vi "TEST - Filter 1D Array.vi"(8 "error in (no error)":errorcluster) -> (0 "error out":errorcluster, 2 "Pass?":bool)   [LabVIEW 2009]
doc: "This VI template can be used for the functional testing of VIs; this implementation includes handling for the testing of polymorphic VIs, and the polymorphic elements should be removed if not needed.\n\nCoded by Douglas A. Femec, January 24, 2006.\n\nCopyright (c) 2005-2006 MKS Instruments, Inc.\nAll rights reserved."
uses:
  TEST - Filter 1D Array - Inputs.ctl
  Polymorphizer+ Data Type.ctl
  TEST - Filter 1D Array - Outputs.ctl
  source/library/Filter 1D Array/Filter 1D Array (EXT).vi
  source/library/Filter 1D Array/Filter 1D Array with Scalar (EXT).vi
  source/library/Filter 1D Array/Filter 1D Array (DBL).vi
  source/library/Filter 1D Array/Filter 1D Array with Scalar (DBL).vi
  source/library/Filter 1D Array/Filter 1D Array with Scalar (LVObject).vi
  source/library/Filter 1D Array/Filter 1D Array (LVObject).vi
  source/library/Filter 1D Array/Filter 1D Array (I64).vi
  source/library/Filter 1D Array/Filter 1D Array with Scalar (I64).vi
  source/library/Filter 1D Array/Filter 1D Array (U64).vi
  source/library/Filter 1D Array/Filter 1D Array with Scalar (U64).vi
  source/library/Filter 1D Array/Filter 1D Array (SGL).vi
  source/library/Filter 1D Array/Filter 1D Array with Scalar (SGL).vi
  source/library/Filter 1D Array/Filter 1D Array (I32).vi
  source/library/Filter 1D Array/Filter 1D Array with Scalar (I32).vi
  source/library/Filter 1D Array/Filter 1D Array (I16).vi
  source/library/Filter 1D Array/Filter 1D Array with Scalar (I16).vi
  source/library/Filter 1D Array/Filter 1D Array (I8).vi
  source/library/Filter 1D Array/Filter 1D Array with Scalar (I8).vi
  source/library/Filter 1D Array/Filter 1D Array (U32).vi
  source/library/Filter 1D Array/Filter 1D Array with Scalar (U32).vi
  source/library/Filter 1D Array/Filter 1D Array (U16).vi
  source/library/Filter 1D Array/Filter 1D Array with Scalar (U16).vi
  source/library/Filter 1D Array/Filter 1D Array (U8).vi
  source/library/Filter 1D Array/Filter 1D Array with Scalar (U8).vi
  source/library/Filter 1D Array/Filter 1D Array (CXT).vi
  source/library/Filter 1D Array/Filter 1D Array with Scalar (CXT).vi
  source/library/Filter 1D Array/Filter 1D Array (CDB).vi
  source/library/Filter 1D Array/Filter 1D Array with Scalar (CDB).vi
  source/library/Filter 1D Array/Filter 1D Array (CSG).vi
  source/library/Filter 1D Array/Filter 1D Array with Scalar (CSG).vi
  source/library/Filter 1D Array/Filter 1D Array (Boolean).vi
  source/library/Filter 1D Array/Filter 1D Array with Scalar (Boolean).vi
  source/library/Filter 1D Array/Filter 1D Array (String).vi
  source/library/Filter 1D Array/Filter 1D Array with Scalar (String).vi
  source/library/Filter 1D Array/Filter 1D Array (Path).vi
  source/library/Filter 1D Array/Filter 1D Array with Scalar (Path).vi
  source/library/Filter 1D Array/Filter 1D Array (Variant).vi
  source/library/Filter 1D Array/Filter 1D Array with Scalar (Variant).vi
  TestClass/TestClass.lvclass
panel:
  out "Generated Outputs":T1[][](array[typedef]) {"Filtered Array (Scalar)" format="%.2f"; "Filtered Array" format="%.2f"}
  in  "Expected Outputs":T1[](array[typedef])=[{"Description"="Expect empty array", "Filtered Array"=[], "Filtered Array (Scalar)"=[]}, {"Description"="Expect no elements filtered", "Filtered Array"=[0.0, 0.0, 0.0, 0.0], "Filtered Array (Scalar)"=[0.0, 0.0, 0.0, 0.0]}, {"Description"="Expect some elements filtered", "Filtered Array"=[0.0, 0.0], "Filtered Array (Scalar)"=[0.0, 0.0]}, {"Description"="Expect all elements filtered", "Filtered Array"=[], "Filtered Array (Scalar)"=[1.0, 1.0]}, {"Description"="Expect all elements filtered", "Filtered Array"=[], "Filtered Array (Scalar)"=[1.0, 1.0]}, {"Description"="Expect all elements filtered", "Filtered Array"=[], "Filtered Array (Scalar)"=[1.0, 1.0]}, {"Description"="Expect all elements filtered", "Filtered Array"=[], "Filtered Array (Scalar)"=[1.0, 1.0]}, {"Description"="Expect all elements filtered", "Filtered Array"=[], "Filtered Array (Scalar)"=[1.0, 1.0]}, {"Description"="Expect all elements filtered", "Filtered Array"=[], "Filtered Array (Scalar)"=[1.0, 1.0]}, {"Description"="Expect all elements filtered", "Filtered Array"=[], "Filtered Array (Scalar)"=[]}, {"Description"="Expect some elements filtered", "Filtered Array"=[0.0, 0.0], "Filtered Array (Scalar)"=[1.0, 1.0]}, {"Description"="Expect some elements filtered", "Filtered Array"=[1.0, 1.0], "Filtered Array (Scalar)"=[1.0, 1.0]}] {"Filtered Array (Scalar)" format="%.2f"; "Filtered Array" format="%.2f"}
  in  "Inputs":T2[](array[typedef])=[{"Description"="Empty arrays", "Data Types to Test"=[enum."EXT", enum."DBL", enum."SGL", enum."I32", enum."I16", enum."I8", enum."U32", enum."U16", enum."U8", enum."CXT", enum."CDB", enum."CSG", enum."Boolean", enum."String", enum."Path", enum."Variant", enum."I64", enum."U64", enum."LabVIEW Object"], "Array"=[], "Items to Filter"=[], "Scalar Item to Filter"=0.0}, {"Description"="No element to filter", "Data Types to Test"=[enum."EXT", enum."DBL", enum."SGL", enum."I32", enum."I16", enum."I8", enum."U32", enum."U16", enum."U8", enum."CXT", enum."CDB", enum."CSG", enum."Boolean", enum."String", enum."Path", enum."Variant", enum."I64", enum."U64", enum."LabVIEW Object"], "Array"=[0.0, 0.0, 0.0, 0.0], "Items to Filter"=[1.0], "Scalar Item to Filter"=1.0}, {"Description"="Filter some elements", "Data Types to Test"=[enum."EXT", enum."DBL", enum."SGL", enum."I32", enum."I16", enum."I8", enum."U32", enum."U16", enum."U8", enum."CXT", enum."CDB", enum."CSG", enum."Boolean", enum."String", enum."Path", enum."Variant", enum."I64", enum."U64", enum."LabVIEW Object"], "Array"=[0.0, 1.0, 0.0, 1.0], "Items to Filter"=[1.0], "Scalar Item to Filter"=1.0}, {"Description"="Filter all elements", "Data Types to Test"=[enum."EXT", enum."DBL", enum."SGL", enum."I32", enum."I16", enum."I8", enum."U32", enum."U16", enum."U8", enum."CXT", enum."CDB", enum."CSG", enum."Boolean", enum."String", enum."Path", enum."Variant", enum."I64", enum."U64", enum."LabVIEW Object"], "Array"=[0.0, 1.0, 0.0, 1.0], "Items to Filter"=[0.0, 1.0], "Scalar Item to Filter"=0.0}, {"Description"="Filter all elements with duplicates early in Items to Filter", "Data Types to Test"=[enum."EXT", enum."DBL", enum."SGL", enum."I32", enum."I16", enum."I8", enum."U32", enum."U16", enum."U8", enum."CXT", enum."CDB", enum."CSG", enum."Boolean", enum."String", enum."Path", enum."Variant", enum."I64", enum."U64", enum."LabVIEW Object"], "Array"=[0.0, 1.0, 0.0, 1.0], "Items to Filter"=[0.0, 0.0, 1.0], "Scalar Item to Filter"=0.0}, {"Description"="Filter all elements with duplicates early in Items to Filter", "Data Types to Test"=[enum."EXT", enum."DBL", enum."SGL", enum."I32", enum."I16", enum."I8", enum."U32", enum."U16", enum."U8", enum."CXT", enum."CDB", enum."CSG", enum."Boolean", enum."String", enum."Path", enum."Variant", enum."I64", enum."U64", enum."LabVIEW Object"], "Array"=[0.0, 1.0, 0.0, 1.0], "Items to Filter"=[1.0, 1.0, 0.0], "Scalar Item to Filter"=0.0}, {"Description"="Filter all elements with duplicates late in Items to Filter", "Data Types to Test"=[enum."EXT", enum."DBL", enum."SGL", enum."I32", enum."I16", enum."I8", enum."U32", enum."U16", enum."U8", enum."CXT", enum."CDB", enum."CSG", enum."Boolean", enum."String", enum."Path", enum."Variant", enum."I64", enum."U64", enum."LabVIEW Object"], "Array"=[0.0, 1.0, 0.0, 1.0], "Items to Filter"=[1.0, 0.0, 0.0], "Scalar Item to Filter"=0.0}, {"Description"="Filter all elements with duplicates late in Items to Filter", "Data Types to Test"=[enum."EXT", enum."DBL", enum."SGL", enum."I32", enum."I16", enum."I8", enum."U32", enum."U16", enum."U8", enum."CXT", enum."CDB", enum."CSG", enum."Boolean", enum."String", enum."Path", enum."Variant", enum."I64", enum."U64", enum."LabVIEW Object"], "Array"=[0.0, 1.0, 0.0, 1.0], "Items to Filter"=[0.0, 1.0, 1.0], "Scalar Item to Filter"=0.0}, {"Description"="Filter all elements with duplicates interspersed in Items to Filter", "Data Types to Test"=[enum."EXT", enum."DBL", enum."SGL", enum."I32", enum."I16", enum."I8", enum."U32", enum."U16", enum."U8", enum."CXT", enum."CDB", enum."CSG", enum."Boolean", enum."String", enum."Path", enum."Variant", enum."I64", enum."U64", enum."LabVIEW Object"], "Array"=[0.0, 1.0, 0.0, 1.0], "Items to Filter"=[1.0, 0.0, 1.0], "Scalar Item to Filter"=0.0}, {"Description"="Filter all elements with duplicates interspersed in Items to Filter", "Data Types to Test"=[enum."EXT", enum."DBL", enum."SGL", enum."I32", enum."I16", enum."I8", enum."U32", enum."U16", enum."U8", enum."CXT", enum."CDB", enum."CSG", enum."Boolean", enum."String", enum."Path", enum."Variant", enum."I64", enum."U64", enum."LabVIEW Object"], "Array"=[], "Items to Filter"=[0.0, 1.0, 0.0], "Scalar Item to Filter"=0.0}, {"Description"="Filter all elements with only duplicates in Items to Filter", "Data Types to Test"=[enum."EXT", enum."DBL", enum."SGL", enum."I32", enum."I16", enum."I8", enum."U32", enum."U16", enum."U8", enum."CXT", enum."CDB", enum."CSG", enum."Boolean", enum."String", enum."Path", enum."Variant", enum."I64", enum."U64", enum."LabVIEW Object"], "Array"=[0.0, 1.0, 0.0, 1.0], "Items to Filter"=[1.0, 1.0], "Scalar Item to Filter"=0.0}, {"Description"="Filter all elements with only duplicates in Items to Filter", "Data Types to Test"=[enum."EXT", enum."DBL", enum."SGL", enum."I32", enum."I16", enum."I8", enum."U32", enum."U16", enum."U8", enum."CXT", enum."CDB", enum."CSG", enum."Boolean", enum."String", enum."Path", enum."Variant", enum."I64", enum."U64", enum."LabVIEW Object"], "Array"=[0.0, 1.0, 0.0, 1.0], "Items to Filter"=[0.0, 0.0], "Scalar Item to Filter"=0.0}] {"Scalar Item to Filter" format="%.2f"; "Array" format="%.2f"; "Items to Filter" format="%.2f"}
  # "Copyright (c) 2005-2006 MKS Instruments, Inc.\nAll rights reserved."
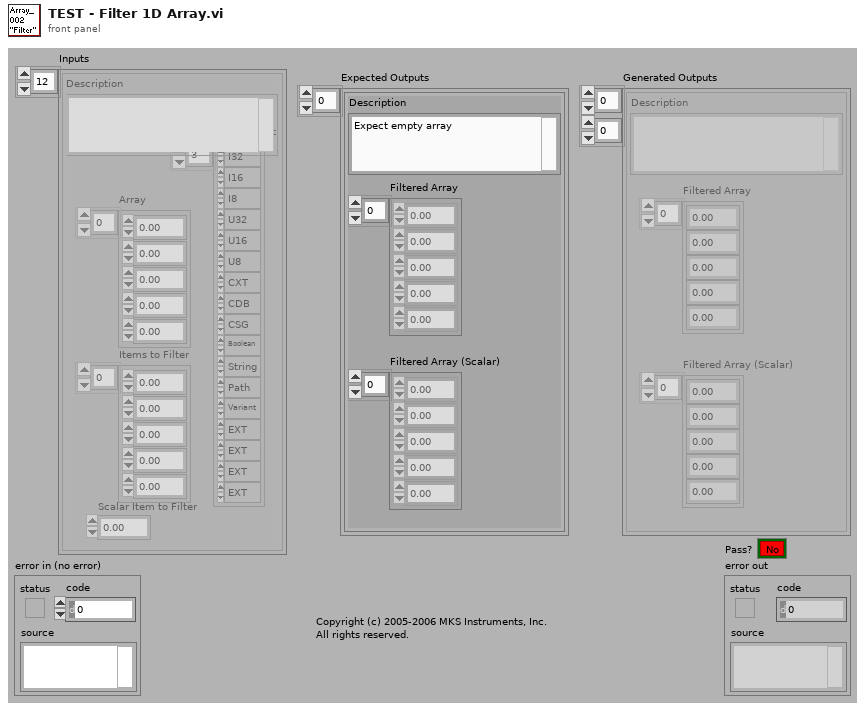
[diagram p1: front panel]
types:
  T1 = typedef "TEST - Filter 1D Array - Outputs.ctl" = cluster{"Description":string, "Filtered Array":sgl[], "Filtered Array (Scalar)":sgl[]}
  T2 = typedef "TEST - Filter 1D Array - Inputs.ctl" = cluster{"Description":string, "Data Types to Test":T3[], "Array":sgl[], "Items to Filter":sgl[], "Scalar Item to Filter":sgl}
  T3 = typedef "Polymorphizer+ Data Type.ctl" = enum16{"EXT", "DBL", "SGL", "I32", "I16", "I8", "U32", "U16", "U8", "CXT", "CDB", "CSG", "Boolean", "String", "Path", "Variant", "CTL-REF", "GEN-REF", "GObj-REF", "VI-REF", "ENUM", "ERR", "FILE-REF", "MENU-REF", "MENU-RING", "PICT-RING", "TXT&PICT-RING", "TXT-RING", "I64", "U64", "LabVIEW Object"}
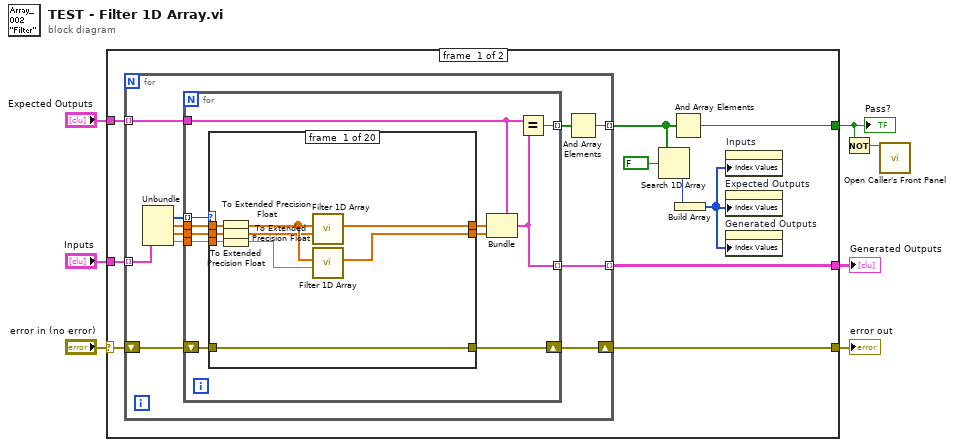
[diagram p0: block diagram]
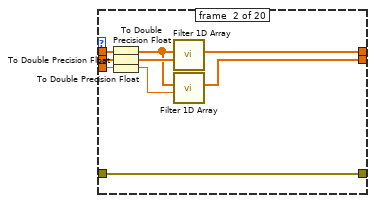
[diagram p2: hidden frame]
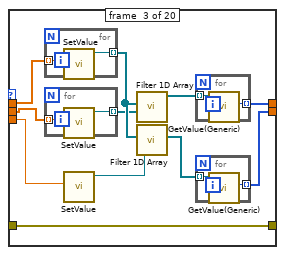
[diagram p3: hidden frame]
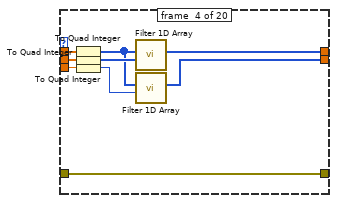
[diagram p4: hidden frame]
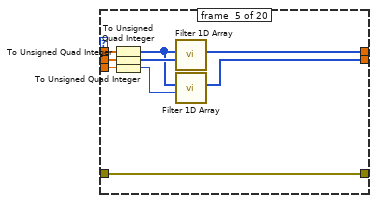
[diagram p5: hidden frame]
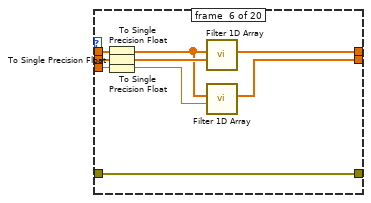
[diagram p6: hidden frame]
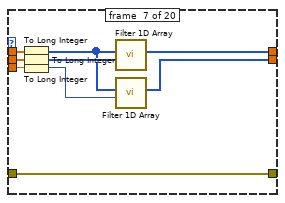
[diagram p7: hidden frame]
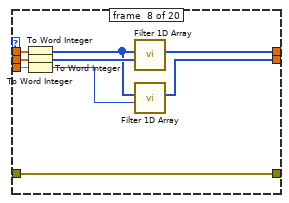
[diagram p8: hidden frame]
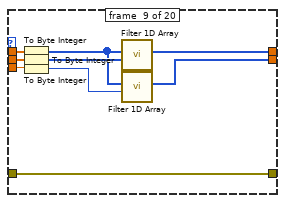
[diagram p9: hidden frame]
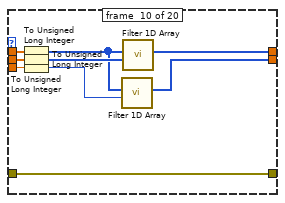
[diagram p10: hidden frame]
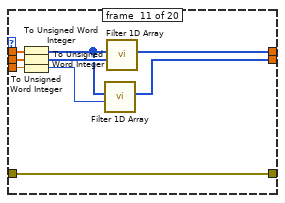
[diagram p11: hidden frame]
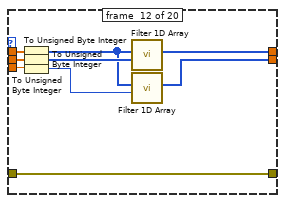
[diagram p12: hidden frame]
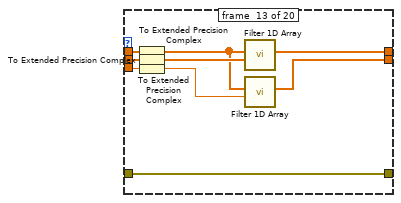
[diagram p13: hidden frame]
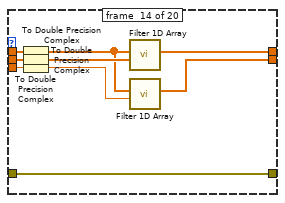
[diagram p14: hidden frame]
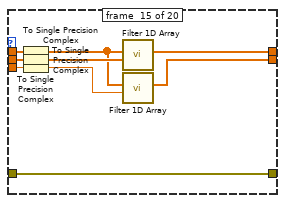
[diagram p15: hidden frame]
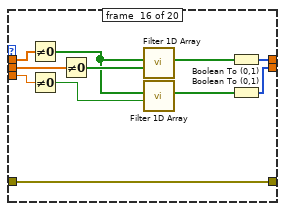
[diagram p16: hidden frame]
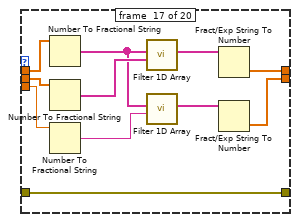
[diagram p17: hidden frame]
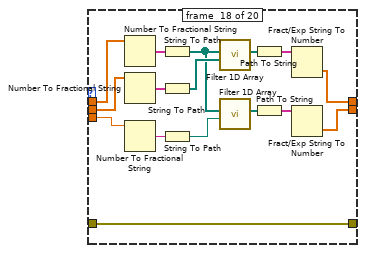
[diagram p18: hidden frame]
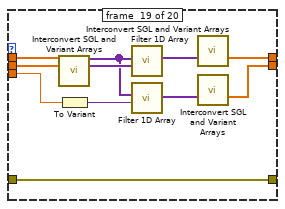
[diagram p19: hidden frame]
diagram:
  n1 = case shown="No Error" "error in (no error)" {
    selector: "error in (no error)" -> [w16 w236]
    tunnel: [w17 w236] -> w6
    tunnel: "Expected Outputs" -> [w14 _]
    tunnel: "Inputs" -> [w15 _]
    tunnel: [w13 _] -> w3
    tunnel: [w12 _] -> w2
    frame #0 {
      n2 = for {
        shift-right: [w23] -> w17
        shift-left: w16 -> [w24]
        tunnel: w15 -> [w25] mode=indexing
        tunnel: w14 -> [w28] mode=indexing
        tunnel: [w27] -> w13 mode=indexing
        tunnel: [w22] -> w11 mode=indexing
        n3 = Unbundle(w25) -> ("Data Types to Test"=w21:T3[], "Array"=w19:sgl[], "Items to Filter"=w20:sgl[], "Scalar Item to Filter"=w18:sgl)  [unwired: 1 out]
        n4 = for {
          tunnel: w28 -> [w39]
          tunnel: [w37] -> w27 mode=indexing
          tunnel: [w38] -> w26 mode=indexing
          shift-right: [w32] -> w23
          shift-left: w24 -> [w33]
          tunnel: w21 -> [w34] mode=indexing
          tunnel: w19 -> [w36]
          tunnel: w20 -> [w35]
          tunnel: w18 -> [w30]
          n5 = case shown="\"LabVIEW Object\"" w34 {
            tunnel: w36 -> [w48 w56 w61 w84 w93 w102 w111 w120 w129 w138 w148 w156 w166 w175 w184 w195 w205 w219 w232 w234]
            tunnel: [w46 w54 w64 w82 w91 w100 w109 w118 w127 w136 w146 w154 w164 w173 w182 w194 w204 w218 w228 w234] -> w31
            tunnel: w35 -> [w43 w57 w58 w85 w94 w103 w112 w121 w130 w139 w143 w157 w159 w168 w177 w190 w206 w221 w231 _]
            tunnel: w33 -> [w47 w55 w68 w83 w92 w101 w110 w119 w128 w137 w147 w155 w165 w174 w183 w193 w203 w216 w233 w235]
            tunnel: [w47 w55 w68 w83 w92 w101 w110 w119 w128 w137 w147 w155 w165 w174 w183 w193 w203 w216 w233 w235] -> w32
            tunnel: w30 -> [w42 w52 w60 w80 w89 w98 w107 w115 w124 w133 w142 w151 w158 w167 w176 w189 w199 w213 w226 _]
            tunnel: [w40 w49 w65 w77 w86 w95 w104 w113 w122 w131 w140 w149 w160 w169 w178 w186 w196 w207 w223 w234] -> w29
            frame #0 {
              n6 = To Extended Precision Float(1:w48) -> (0:w45:ext[])
              n7 = To Extended Precision Float(1:w43) -> (0:w44:ext[])
              n8 = To Extended Precision Float(1:w42) -> (0:w41:ext)
              n9 = call-poly "Filter 1D Array.vi"("items to filter"=w44, "array"=w45) -> ("filtered array"=w46:ext[])  [unwired: 4 in, 1 out]
              n10 = call-poly "Filter 1D Array.vi"("items to filter"=w41, "array"=w45) -> ("filtered array"=w40:ext[])  [unwired: 4 in, 1 out]
            }
            frame #1 {
              n11 = To Double Precision Float(number=w56) -> (double precision float=w50:dbl[])
              n12 = To Double Precision Float(number=w57) -> (double precision float=w53:dbl[])
              n13 = To Double Precision Float(number=w52) -> (double precision float=w51:dbl)
              n14 = call-poly "Filter 1D Array.vi"("items to filter"=w53, "array"=w50) -> ("filtered array"=w54:dbl[])  [unwired: 4 in, 1 out]
              n15 = call-poly "Filter 1D Array.vi"("items to filter"=w51, "array"=w50) -> ("filtered array"=w49:dbl[])  [unwired: 4 in, 1 out]
            }
            frame #2 {
              n16 = for {
                tunnel: [w72] -> w62 mode=indexing
                tunnel: w61 -> [w71] mode=indexing
                n17 = call "SetValue.vi"("Value"=w71) -> ("TestClass out"=w72:refnum<class "TestClass.lvclass">)  [unwired: 9 in, 1 out]
              }
              n18 = for {
                tunnel: [w70] -> w59 mode=indexing
                tunnel: w58 -> [w69] mode=indexing
                n19 = call "SetValue.vi"("Value"=w69) -> ("TestClass out"=w70:refnum<class "TestClass.lvclass">)  [unwired: 9 in, 1 out]
              }
              n20 = call "SetValue.vi"("Value"=w60) -> ("TestClass out"=w67:refnum<class "TestClass.lvclass">)  [unwired: 9 in, 1 out]
              n21 = call-poly "Filter 1D Array.vi"("items to filter"=w59, "array"=w62) -> ("filtered array"=w63:refnum<class>[])  [unwired: 4 in, 1 out]
              n22 = call-poly "Filter 1D Array.vi"("items to filter"=w67, "array"=w62) -> ("filtered array"=w66:refnum<class>[])  [unwired: 4 in, 1 out]
              n23 = for {
                tunnel: w63 -> [w74] mode=indexing
                tunnel: [w73] -> w64 mode=indexing
                n24 = call "GetValue(Generic).vi"("TestClass in"=w74) -> ("Value"=w73:i32)  [unwired: 8 in, 2 out]
              }
              n25 = for {
                tunnel: w66 -> [w76] mode=indexing
                tunnel: [w75] -> w65 mode=indexing
                n26 = call "GetValue(Generic).vi"("TestClass in"=w76) -> ("Value"=w75:i32)  [unwired: 8 in, 2 out]
              }
            }
            frame #3 {
              n27 = To Quad Integer(1:w84) -> (0:w78:i64[])
              n28 = To Quad Integer(1:w85) -> (0:w81:i64[])
              n29 = To Quad Integer(1:w80) -> (0:w79:i64)
              n30 = call-poly "Filter 1D Array.vi"("items to filter"=w81, "array"=w78) -> ("filtered array"=w82:i64[])  [unwired: 4 in, 1 out]
              n31 = call-poly "Filter 1D Array.vi"("items to filter"=w79, "array"=w78) -> ("filtered array"=w77:i64[])  [unwired: 4 in, 1 out]
            }
            frame #4 {
              n32 = To Unsigned Quad Integer(1:w93) -> (0:w87:u64[])
              n33 = To Unsigned Quad Integer(1:w94) -> (0:w90:u64[])
              n34 = To Unsigned Quad Integer(1:w89) -> (0:w88:u64)
              n35 = call-poly "Filter 1D Array.vi"("items to filter"=w90, "array"=w87) -> ("filtered array"=w91:u64[])  [unwired: 4 in, 1 out]
              n36 = call-poly "Filter 1D Array.vi"("items to filter"=w88, "array"=w87) -> ("filtered array"=w86:u64[])  [unwired: 4 in, 1 out]
            }
            frame #5 {
              n37 = To Single Precision Float(number=w102) -> (single precision float=w97:sgl[])
              n38 = To Single Precision Float(number=w103) -> (single precision float=w99:sgl[])
              n39 = To Single Precision Float(number=w98) -> (single precision float=w96:sgl)
              n40 = call-poly "Filter 1D Array.vi"("items to filter"=w99, "array"=w97) -> ("filtered array"=w100:sgl[])  [unwired: 4 in, 1 out]
              n41 = call-poly "Filter 1D Array.vi"("items to filter"=w96, "array"=w97) -> ("filtered array"=w95:sgl[])  [unwired: 4 in, 1 out]
            }
            frame #6 {
              n42 = To Long Integer(number=w111) -> (32bit integer=w105:i32[])
              n43 = To Long Integer(number=w112) -> (32bit integer=w108:i32[])
              n44 = To Long Integer(number=w107) -> (32bit integer=w106:i32)
              n45 = call-poly "Filter 1D Array.vi"("items to filter"=w108, "array"=w105) -> ("filtered array"=w109:i32[])  [unwired: 4 in, 1 out]
              n46 = call-poly "Filter 1D Array.vi"("items to filter"=w106, "array"=w105) -> ("filtered array"=w104:i32[])  [unwired: 4 in, 1 out]
            }
            frame #7 {
              n47 = To Word Integer(number=w120) -> (16bit integer=w114:i16[])
              n48 = To Word Integer(number=w121) -> (16bit integer=w117:i16[])
              n49 = To Word Integer(number=w115) -> (16bit integer=w116:i16)
              n50 = call-poly "Filter 1D Array.vi"("items to filter"=w117, "array"=w114) -> ("filtered array"=w118:i16[])  [unwired: 4 in, 1 out]
              n51 = call-poly "Filter 1D Array.vi"("items to filter"=w116, "array"=w114) -> ("filtered array"=w113:i16[])  [unwired: 4 in, 1 out]
            }
            frame #8 {
              n52 = To Byte Integer(number=w129) -> (8bit integer=w125:i8[])
              n53 = To Byte Integer(number=w130) -> (8bit integer=w126:i8[])
              n54 = To Byte Integer(number=w124) -> (8bit integer=w123:i8)
              n55 = call-poly "Filter 1D Array.vi"("items to filter"=w126, "array"=w125) -> ("filtered array"=w127:i8[])  [unwired: 4 in, 1 out]
              n56 = call-poly "Filter 1D Array.vi"("items to filter"=w123, "array"=w125) -> ("filtered array"=w122:i8[])  [unwired: 4 in, 1 out]
            }
            frame #9 {
              n57 = To Unsigned Long Integer(number=w138) -> (unsigned 32bit integer=w134:u32[])
              n58 = To Unsigned Long Integer(number=w139) -> (unsigned 32bit integer=w135:u32[])
              n59 = To Unsigned Long Integer(number=w133) -> (unsigned 32bit integer=w132:u32)
              n60 = call-poly "Filter 1D Array.vi"("items to filter"=w132, "array"=w134) -> ("filtered array"=w131:u32[])  [unwired: 4 in, 1 out]
              n61 = call-poly "Filter 1D Array.vi"("items to filter"=w135, "array"=w134) -> ("filtered array"=w136:u32[])  [unwired: 4 in, 1 out]
            }
            frame #10 {
              n62 = To Unsigned Word Integer(number=w148) -> (unsigned 16bit integer=w144:u16[])
              n63 = To Unsigned Word Integer(number=w143) -> (unsigned 16bit integer=w145:u16[])
              n64 = To Unsigned Word Integer(number=w142) -> (unsigned 16bit integer=w141:u16)
              n65 = call-poly "Filter 1D Array.vi"("items to filter"=w141, "array"=w144) -> ("filtered array"=w140:u16[])  [unwired: 4 in, 1 out]
              n66 = call-poly "Filter 1D Array.vi"("items to filter"=w145, "array"=w144) -> ("filtered array"=w146:u16[])  [unwired: 4 in, 1 out]
            }
            frame #11 {
              n67 = To Unsigned Byte Integer(number=w156) -> (unsigned 8bit integer=w152:u8[])
              n68 = To Unsigned Byte Integer(number=w157) -> (unsigned 8bit integer=w153:u8[])
              n69 = To Unsigned Byte Integer(number=w151) -> (unsigned 8bit integer=w150:u8)
              n70 = call-poly "Filter 1D Array.vi"("items to filter"=w153, "array"=w152) -> ("filtered array"=w154:u8[])  [unwired: 4 in, 1 out]
              n71 = call-poly "Filter 1D Array.vi"("items to filter"=w150, "array"=w152) -> ("filtered array"=w149:u8[])  [unwired: 4 in, 1 out]
            }
            frame #12 {
              n72 = To Extended Precision Complex(1:w166) -> (0:w162:cxt[])
              n73 = To Extended Precision Complex(1:w159) -> (0:w163:cxt[])
              n74 = To Extended Precision Complex(1:w158) -> (0:w161:cxt)
              n75 = call-poly "Filter 1D Array.vi"("items to filter"=w163, "array"=w162) -> ("filtered array"=w164:cxt[])  [unwired: 4 in, 1 out]
              n76 = call-poly "Filter 1D Array.vi"("items to filter"=w161, "array"=w162) -> ("filtered array"=w160:cxt[])  [unwired: 4 in, 1 out]
            }
            frame #13 {
              n77 = To Double Precision Complex(1:w175) -> (0:w171:cdb[])
              n78 = To Double Precision Complex(1:w168) -> (0:w172:cdb[])
              n79 = To Double Precision Complex(1:w167) -> (0:w170:cdb)
              n80 = call-poly "Filter 1D Array.vi"("items to filter"=w172, "array"=w171) -> ("filtered array"=w173:cdb[])  [unwired: 4 in, 1 out]
              n81 = call-poly "Filter 1D Array.vi"("items to filter"=w170, "array"=w171) -> ("filtered array"=w169:cdb[])  [unwired: 4 in, 1 out]
            }
            frame #14 {
              n82 = To Single Precision Complex(1:w184) -> (0:w180:csg[])
              n83 = To Single Precision Complex(1:w177) -> (0:w181:csg[])
              n84 = To Single Precision Complex(1:w176) -> (0:w179:csg)
              n85 = call-poly "Filter 1D Array.vi"("items to filter"=w181, "array"=w180) -> ("filtered array"=w182:csg[])  [unwired: 4 in, 1 out]
              n86 = call-poly "Filter 1D Array.vi"("items to filter"=w179, "array"=w180) -> ("filtered array"=w178:csg[])  [unwired: 4 in, 1 out]
            }
            frame #15 {
              n87 = Not Equal To 0?(x=w195) -> (x != 0?=w188:bool[])
              n88 = Not Equal To 0?(x=w189) -> (x != 0?=w187:bool)
              n89 = Not Equal To 0?(x=w190) -> (x != 0?=w191:bool[])
              n90 = call-poly "Filter 1D Array.vi"("items to filter"=w191, "array"=w188) -> ("filtered array"=w192:bool[])  [unwired: 4 in, 1 out]
              n91 = call-poly "Filter 1D Array.vi"("items to filter"=w187, "array"=w188) -> ("filtered array"=w185:bool[])  [unwired: 4 in, 1 out]
              n92 = Boolean To (0,1)(Boolean=w192) -> (0, 1=w194:i16[])
              n93 = Boolean To (0,1)(Boolean=w185) -> (0, 1=w186:i16[])
            }
            frame #16 {
              n94 = Number To Fractional String(number=w205) -> (F-format string=w200:string[])  [unwired: 3 in]
              n95 = Number To Fractional String(number=w206) -> (F-format string=w201:string[])  [unwired: 3 in]
              n96 = Number To Fractional String(number=w199) -> (F-format string=w198:string)  [unwired: 3 in]
              n97 = call-poly "Filter 1D Array.vi"("items to filter"=w201, "array"=w200) -> ("filtered array"=w202:string[])  [unwired: 4 in, 1 out]
              n98 = call-poly "Filter 1D Array.vi"("items to filter"=w198, "array"=w200) -> ("filtered array"=w197:string[])  [unwired: 4 in, 1 out]
              n99 = Fract/Exp String To Number(string=w202) -> (number=w204:dbl[])  [unwired: 3 in, 1 out]
              n100 = Fract/Exp String To Number(string=w197) -> (number=w196:dbl[])  [unwired: 3 in, 1 out]
            }
            frame #17 {
              n101 = Number To Fractional String(number=w219) -> (F-format string=w220:string[])  [unwired: 3 in]
              n102 = Number To Fractional String(number=w221) -> (F-format string=w222:string[])  [unwired: 3 in]
              n103 = Number To Fractional String(number=w213) -> (F-format string=w214:string)  [unwired: 3 in]
              n104 = String To Path(string=w220) -> (path=w211:path[])
              n105 = String To Path(string=w222) -> (path=w212:path[])
              n106 = String To Path(string=w214) -> (path=w210:path)
              n107 = call-poly "Filter 1D Array.vi"("items to filter"=w212, "array"=w211) -> ("filtered array"=w215:path[])  [unwired: 4 in, 1 out]
              n108 = call-poly "Filter 1D Array.vi"("items to filter"=w210, "array"=w211) -> ("filtered array"=w208:path[])  [unwired: 4 in, 1 out]
              n109 = Path To String(path=w215) -> (string=w217:string[])
              n110 = Path To String(path=w208) -> (string=w209:string[])
              n111 = Fract/Exp String To Number(string=w217) -> (number=w218:dbl[])  [unwired: 3 in, 1 out]
              n112 = Fract/Exp String To Number(string=w209) -> (number=w207:dbl[])  [unwired: 3 in, 1 out]
            }
            frame #18 {
              n113 = call "Interconvert SGL and Variant Arrays.vi"("SGL 1D Array In"=w232, "SGL 1D Array 2 In"=w231) -> ("Variant 1D Array Out"=w227:variant[], "Variant 1D Array 2 Out"=w230:variant[])  [unwired: 9 in, 3 out]
              n114 = To Variant(anything=w226) -> (Variant=w225:variant)
              n115 = call-poly "Filter 1D Array.vi"("items to filter"=w230, "array"=w227) -> ("filtered array"=w229:variant[])  [unwired: 4 in, 1 out]
              n116 = call-poly "Filter 1D Array.vi"("items to filter"=w225, "array"=w227) -> ("filtered array"=w224:variant[])  [unwired: 4 in, 1 out]
              n117 = call "Interconvert SGL and Variant Arrays.vi"("Variant 1D Array In"=w229) -> ("SGL 1D Array Out"=w228:sgl[])  [unwired: 10 in, 4 out]
              n118 = call "Interconvert SGL and Variant Arrays.vi"("Variant 1D Array In"=w224) -> ("SGL 1D Array Out"=w223:sgl[])  [unwired: 10 in, 4 out]
            }
            frame #19 {
            }
          }
          n119 = Bundle(cluster=w39, "Filtered Array"=w31, "Filtered Array (Scalar)"=w29) -> (w37:T1)  [unwired: 1 in]
          n120 = Equal?(x=w39, y=w37) -> (x = y?=w38:bool)
        }
        n121 = And Array Elements(Boolean array=w26) -> (logical AND=w22:bool)
      }
      n122 = Search 1D Array(1D array=w11, element=FALSE) -> (index of element=w9:i32)  [unwired: 1 in]
      n123 = And Array Elements(Boolean array=w11) -> (logical AND=w12:bool)
      n124 = Build Array(w9) -> (w8:i32[])
      n125 = property on="Inputs" class="Arr (strict)"("Index Values"=w8) -> ()  [unwired: 2 in, 2 out]
      n126 = property on="Expected Outputs" class="Arr (strict)"("Index Values"=w8) -> ()  [unwired: 2 in, 2 out]
      n127 = property on="Generated Outputs" class="Arr (strict)"("Index Values"=w8) -> ()  [unwired: 2 in, 2 out]
    }
    frame #1 {
    }
  }
  "error out" <- w6
  "Pass?" <- w2
  "Generated Outputs" <- w3
  n128 = Not(x=w2) -> (.not. x?=w1:bool)
  n129 = call "Open Caller's Front Panel.vi"("Open?"=w1) -> ()  [unwired: 14 in, 1 out]
